vi "init.vi"(8 "error in":errorcluster, 10 "TBM module configuration in":refnum<class "TBM module configuration.lvclass">, 11 "Profibus Module runtime in":refnum<class "Profibus Module runtime.lvclass">) -> (0 "error out":errorcluster, 1 "data allocations":T1, 2 "execution settings":T4, 3 "Profibus Module runtime out":refnum<class "Profibus Module runtime.lvclass">)   [LabVIEW 2013, in "Profibus Module runtime.lvclass"]
doc: "Provides an interface for initializing a module at runtime. While this interface performs no operations, a child should provide an override which may open any necessary references or sessions, allocate necessary memory, and perform any final configuration validataion before providing the full configuration <b>execution data</b> to the calling process."
uses:
  Profibus Module runtime.lvclass
  <vilib>/NI/Tag Bus Module Framework/channel/TBM channel.lvclass
  <vilib>/NI/Tag Bus Module Framework/runtime/TBM module execution interface.lvclass
  configuration/Profibus Module configuration.lvclass
  dynamic profibus/dynamic profibus.lvlib
  dynamic profibus/CS_cRIO-PB_DP-Master_FPGA-Reference.ctl
  <vilib>/NI/Tag Bus Module Framework/FPGA manager/FPGA manager.lvlib
  <vilib>/NI/Tag Bus Module Framework/FPGA manager/methods.ctl
  <vilib>/NI/Tag Bus Module Framework/module configuration/TBM module configuration.lvclass
  <vilib>/NI/Tag Bus Module Framework/runtime/execution settings.ctl
  <vilib>/NI/Tag Bus Module Framework/channel/data tables.ctl
  <vilib>/NI/Tag Bus/dictionary/data dictionary.lvclass
  <vilib>/NI/Tag Bus/dictionary table pair.ctl
  <vilib>/NI/Tag Bus/tag bus.lvlib
  <vilib>/NI/Tag Bus/table/data table.ctl
  <vilib>/NI/Tag Bus/table/data table.lvlib
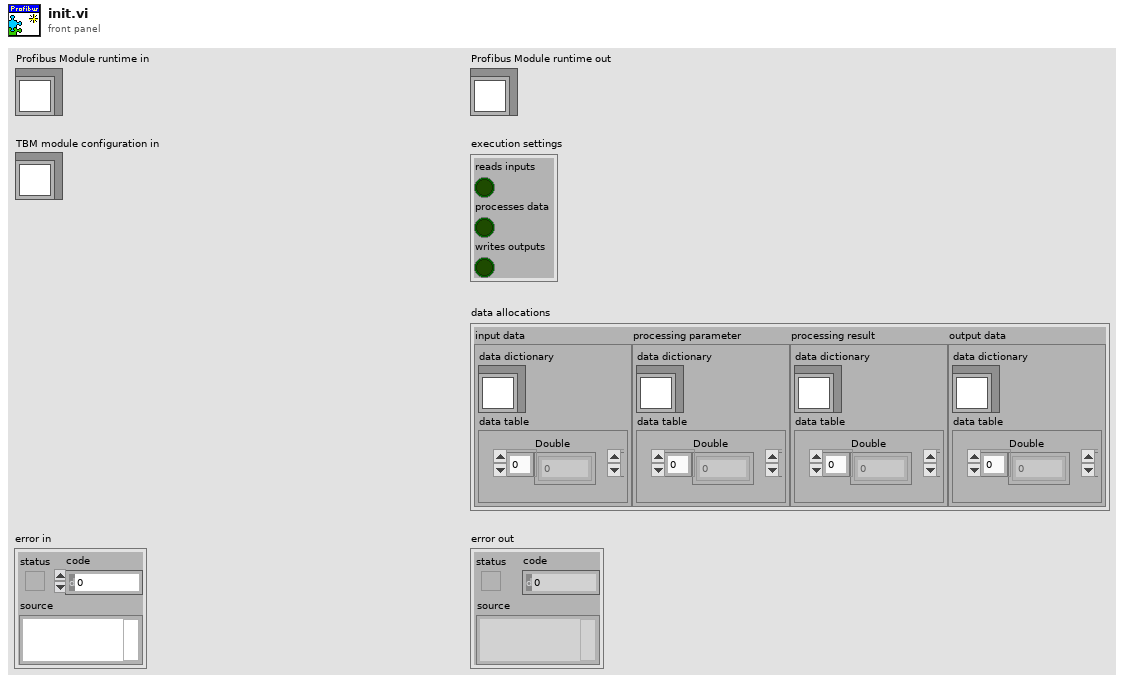
[diagram p1: front panel]
types:
  T1 = typedef "TBM channel.lvclass/data tables.ctl" = cluster{"input data":T2, "processing parameter":T2, "processing result":T2, "output data":T2}
  T2 = typedef "tag bus.lvlib/dictionary table pair.ctl" = cluster{"data dictionary":refnum<class "data dictionary.lvclass">, "data table":T3}
  T3 = typedef "tag bus.lvlib/data table.lvlib/data table.ctl" = cluster{"Double":dbl[], "Single":sgl[], "I64":i64[], "I32":i32[], "I16":i16[], "I8":i8[], "U64":u64[], "U32":u32[], "U16":u16[], "U8":u8[], "Boolean":bool[], "String":string[], "Array of Double":cluster{"DBL Array":dbl[]}[], "Array of Single":cluster{"SGL Array":sgl[]}[], "Array of I64":cluster{"I64 Array":i64[]}[], "Array of I32":cluster{"I32 Array":i32[]}[], "Array of I16":cluster{"I16 Array":i16[]}[], "Array of I8":cluster{"I8 Array":i8[]}[], "Array of U64":cluster{"U64 Array":u64[]}[], "Array of U32":cluster{"U32 Array":u32[]}[], "Array of U16":cluster{"U16 Array":u16[]}[], "Array of U8":cluster{"U8 Array":u8[]}[], "Array of Boolean":cluster{"Boolean Array":bool[]}[], "Array of String":cluster{"String Array":string[]}[]}
  T4 = typedef "TBM module execution interface.lvclass/execution settings.ctl" = cluster{"reads inputs":bool, "processes data":bool, "writes outputs":bool}
  T5 = typedef "FPGA manager.lvlib/methods.ctl" = enum16{"initialize bitfile", "cache bitfile", "locate bitfile", "close bitfile"}
  T6 = typedef "dynamic profibus.lvlib/CS_cRIO-PB_DP-Master_FPGA-Reference.ctl" = refnum<k20>
  T7 = cluster{"Address":i8, "Input Length":u8, "Output Length":u8}[]
  T8 = typedef "Profibus Module runtime.lvclass/profibus diagnostics reporting.ctl" = cluster{"slave":i8, "report":bool, "diagnostic tag":i32, "error specs":T9[]}
  T9 = typedef "Profibus Module configuration.lvclass/error throw specification.ctl" = cluster{"byte":i32, "bit":i32, "inverted?":bool, "error":i32}
  T10 = typedef "Profibus Module runtime.lvclass/profibus slave configuration.ctl" = cluster{"slave index":i8, "data items":T11[], "data buffer":u8[], "big endian":bool, "data length":i32}
  T11 = typedef "Profibus Module runtime.lvclass/profibus mapping configuration.ctl" = cluster{"data type":T12, " byte":i32, " bit":i32, "tag index":i32}
  T12 = typedef "tag bus.lvlib/tag descriptor.lvclass/Data Type.ctl" = enum16{"Double", "Single", "I64", "I32", "I16", "I8", "U64", "U32", "U16", "U8", "Boolean", "String", "Array of Double", "Array of Single", "Array of I64", "Array of I32", "Array of I16", "Array of I8", "Array of U64", "Array of U32", "Array of U16", "Array of U8", "Array of Boolean", "Array of String"}
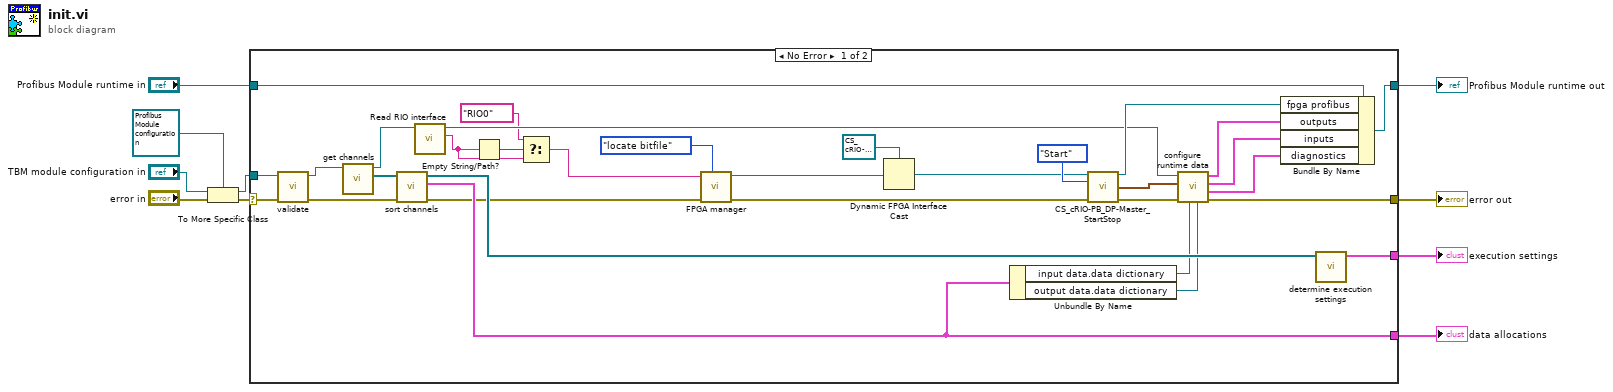
[diagram p0: block diagram]
diagram:
  n1 = To More Specific Class(target class=refnum<class "Profibus Module configuration.lvclass"> refnum ("Synchronous module configuration"), reference="TBM module configuration in", error in="error in") -> (specific class reference=w9:refnum<class "Profibus Module configuration.lvclass">, error out=w10:errorcluster)
  n2 = case shown="No Error" w10 {
    selector: w10 -> [w38 w43]
    tunnel: w9 -> [w37 _]
    tunnel: "Profibus Module runtime in" -> [w42 w44]
    tunnel: [w34 w44] -> w4
    tunnel: [w29 w43] -> w3
    tunnel: [w27 _] -> w1
    tunnel: [w41 _] -> w2
    frame No Error {
      n3 = call-dynamic "validate.vi"("error in"=w38, "Profibus Module configuration in"=w37) -> ("error out"=w39:errorcluster, "Profibus Module configuration out"=w36:refnum<class "Profibus Module configuration.lvclass">)  [unwired: 8 in]
      n4 = call-dynamic "get channels.vi"("Profibus Module configuration in"=w36) -> ("channels"=w35:refnum<class "TBM channel.lvclass">[], "Profibus Module configuration out"=w20:refnum<class "Profibus Module configuration.lvclass">)  [unwired: 9 in]
      n5 = call <vilib>:"sort channels.vi"("error in"=w39, "channels in"=w35) -> ("error out"=w16:errorcluster, "data allocations"=w27:T1, "channels out"=w40:refnum<class "TBM channel.lvclass">[])  [unwired: 7 in]
      n6 = call "Read RIO interface.vi"("Profibus Module configuration in"=w20) -> ("RIO interface"=w17:string, "Profibus Module configuration out"=w21:refnum<class "Profibus Module configuration.lvclass">)  [unwired: 8 in, 1 out]
      n7 = Empty String/Path?(string/path=w17) -> (empty?=w19:bool)
      n8 = Select(t=tag "RIO0" ("resource name"), s=w19, f=w17) -> (s? t:f=w13:string)
      n9 = call <vilib>:"FPGA manager.vi"("action"=methods."locate bitfile", "error in"=w16, "RIO resource"=w13) -> ("error out"=w14:errorcluster, "bitfile"=w15:refnum<k20>)  [unwired: 6 in, 1 out]
      n10 = Dynamic FPGA Interface Cast(Session In=T6 refnum ("profibus reference"), Type=w15) -> (Session Out=w23:T6)
      n11 = Unbundle By Name(w27) -> ("input data.data dictionary"=w25:refnum<class "data dictionary.lvclass">, "output data.data dictionary"=w26:refnum<class "data dictionary.lvclass">)
      n12 = call "CS_cRIO-PB_DP-Master_StartStop.vi"("FPGA VI Reference"=w23, "DP-Master"=enum16{"Start", "Stop"}."Start", "Error"=w14) -> ("FPGA VI Reference out"=w22:T6, "Slave Info List"=w28:T7, "Error out"=w30:errorcluster)  [unwired: 10 in]
      n13 = call "configure runtime data.vi"("output dictionary"=w26, "input dictionary"=w25, "error in"=w30, "Slave Info List"=w28, "Profibus Module configuration in"=w21) -> ("error out"=w29:errorcluster, "diagnostics"=w11:T8[], "inputs"=w31:T10[], "outputs"=w32:T10[])  [unwired: 3 in]
      n14 = Bundle By Name(cluster=w42, "fpga profibus"=w22, "outputs"=w32, "inputs"=w31, "diagnostics"=w11) -> (w34:refnum<class "Profibus Module runtime.lvclass">)
      n15 = call <vilib>:"determine execution settings.vi"("channels"=w40) -> ("execution settings"=w41:T4)  [unwired: 10 in]
    }
    frame Error {
    }
  }
  "error out" <- w3
  "Profibus Module runtime out" <- w4
  "execution settings" <- w2
  "data allocations" <- w1
